vi "set frequncy for up converter.vi"(8 "error in (no error)":errorcluster, 11 "p2p vst in":refnum<class "p2p vst.lvclass">) -> (0 "error out":errorcluster, 3 "p2p vst out":refnum<class "p2p vst.lvclass">)   [LabVIEW 2021, in "p2p vst.lvclass"]
uses:
  p2p vst.lvclass
  p2p vst.lvclass/p2p vst.ctl
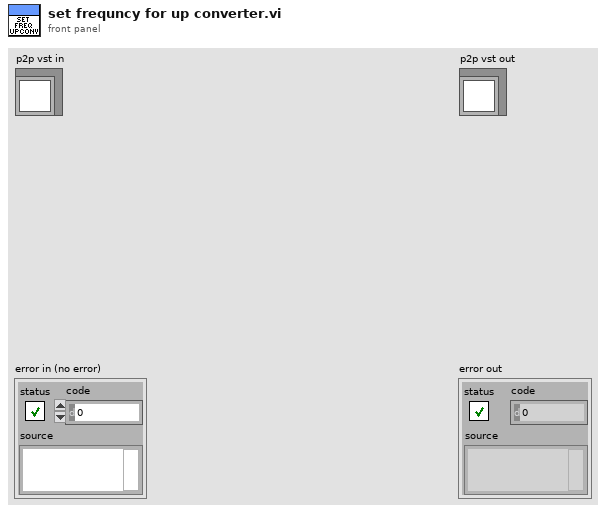
[diagram p1: front panel]
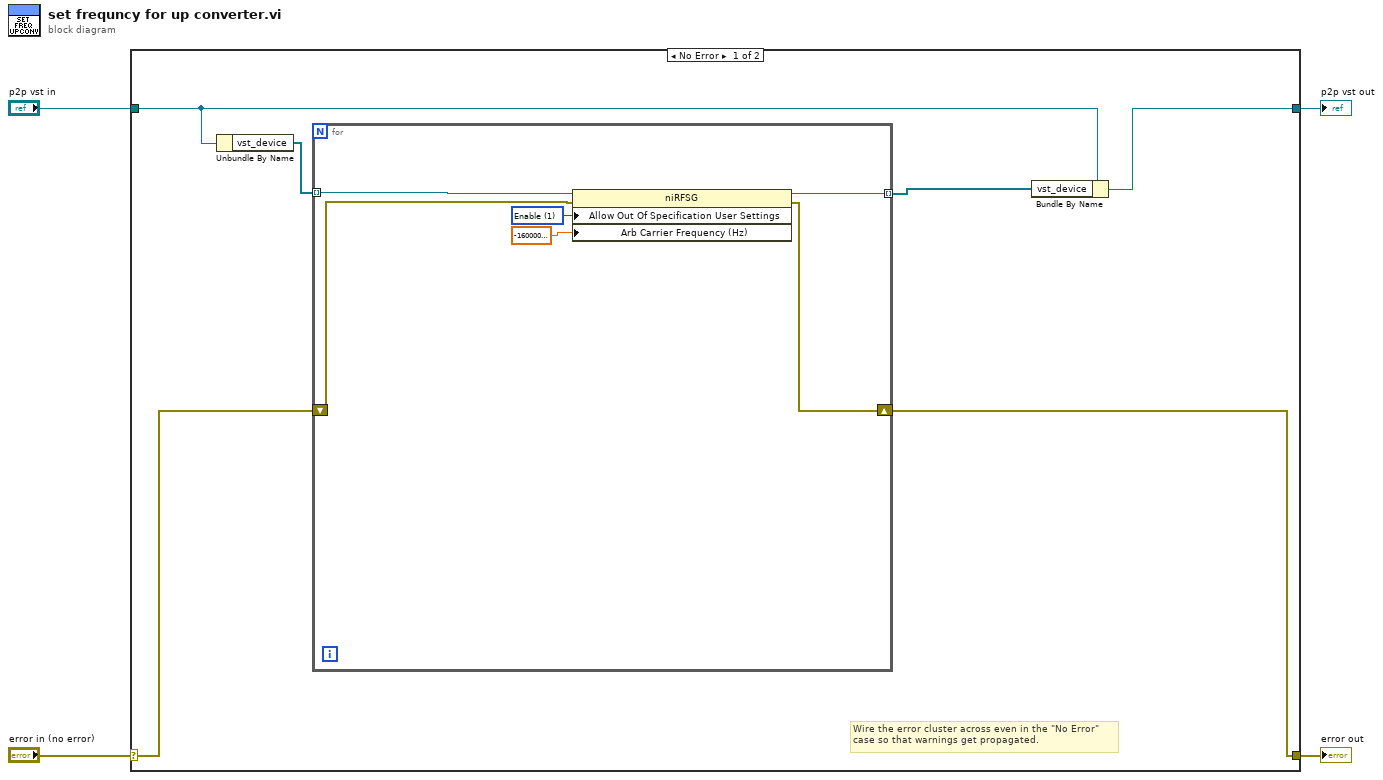
[diagram p0: block diagram]
diagram:
  n1 = case shown="No Error" "error in (no error)" {
    selector: "error in (no error)" -> [w9 w18]
    tunnel: [w5 w18] -> w3
    tunnel: [w6 w17] -> w1
    tunnel: "p2p vst in" -> [w8 w17]
    frame No Error {
      # "Wire the error cluster across even in the \"No Error\"\ncase so that warnings get propagated."
      n2 = Unbundle By Name(w8) -> ("vst_device"=w10:refnum<k15>[])
      n3 = for {
        tunnel: w10 -> [w16] mode=indexing
        shift-right: [w12] -> w5
        shift-left: w9 -> [w13]
        tunnel: [w11] -> w7 mode=indexing
        w15 = 1 items=["Disable", "Enable"] ("RF:Allow Out Of Specification User Settings")
        n4 = property class="niRFSG"(reference=w16, error in=w13, "Allow Out Of Specification User Settings"=w15, "Arb Carrier Frequency (Hz)"=-160000000.0 ("RF:LO Frequency (Hz)")) -> (reference out=w11:refnum<k15>, error out=w12:errorcluster)
      }
      n5 = Bundle By Name(cluster=w8, "vst_device"=w7) -> (w6:refnum<class "p2p vst.lvclass">)
    }
    frame Error {
    }
  }
  "error out" <- w3
  "p2p vst out" <- w1
